vi "Destructor.vi"(8 "error in":errorcluster, 11 "DateTimeMeasureLimit":refnum<class "DateTimeMeasureLimit.lvclass">) -> (0 "error out":errorcluster)   [LabVIEW 2021, in "ProligentXMLGenerator.lvlib" / "DateTimeMeasureLimit.lvclass"]
uses:
  DateTimeMeasureLimit.lvclass
  DateTimeMeasureLimit.lvclass/DateTimeMeasureLimit.ctl
  MeasureLimit/MeasureLimit.lvclass
  RangeMeasureLimit/RangeMeasureLimit.lvclass
  C:/Projects/proligent-xml-generator-labview/src/ProligentXMLGenerator/Measure/RangeMeasureLimit/RangeMeasureLimit.lvclass
  C:/Projects/proligent-xml-generator-labview/src/ProligentXMLGenerator/Measure/MeasureLimit/MeasureLimit.lvclass
  C:/Projects/proligent-xml-generator-labview/src/ProligentXMLGenerator/Measure/DateTimeMeasureLimit/DateTimeMeasureLimit.lvclass
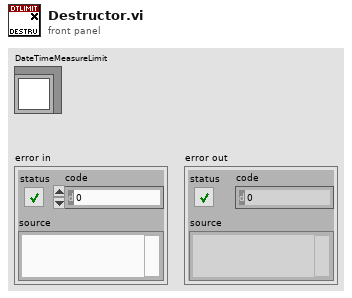
[diagram p1: front panel]
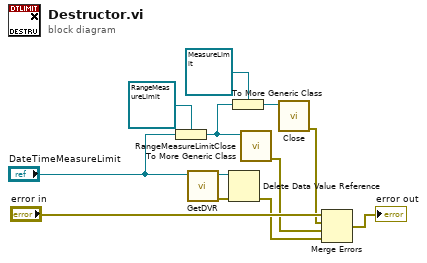
[diagram p0: block diagram]
diagram:
  n1 = To More Generic Class(target class=refnum<class "RangeMeasureLimit.lvclass"> refnum ("ProligentResultProcessor:RangeMeasureLimit"), reference="DateTimeMeasureLimit") -> (generic class reference=w4:refnum<class "RangeMeasureLimit.lvclass">)
  n2 = call "GetDVR.vi"("DateTimeMeasureLimit"="DateTimeMeasureLimit") -> ("error out"=w9:errorcluster, "DVRReference"=w10:refnum<data-value>)  [unwired: 9 in]
  n3 = Delete Data Value Reference(data value reference=w10, error in=w9) -> (error out=w8:errorcluster)  [unwired: 1 out]
  n4 = To More Generic Class(target class=refnum<class "MeasureLimit.lvclass"> refnum ("ProligentResultProcessor:MeasureLimit"), reference=w4) -> (generic class reference=w5:refnum<class "MeasureLimit.lvclass">)
  n5 = call "RangeMeasureLimitClose.vi"("RangeMeasureLimit"=w4) -> ("error out"=w3:errorcluster)  [unwired: 10 in]
  n6 = call "Close.vi"("MeasureLimit"=w5) -> ("error out"=w2:errorcluster)  [unwired: 10 in]
  n7 = Merge Errors("error in", w2, w3, w8) -> (→"error out":errorcluster)
